vi "Mecanum Angular Drift Correction.vi"(1 "Reset":bool, 3 "Gyro":dbl, 6 "Joystick Rotation":dbl) -> (0 "Mecanum Rotation":dbl)   [LabVIEW 2014]
uses:
  <vilib>/addons/control/pid/pid.llb/PID (DBL).vi
  <vilib>/addons/control/pid/NI_PID_pid.lvlib
panel:
  in  "PID gains":T1={"proportional gain (Kc)"=1.0, "integral time (Ti, min)"=0.01, "derivative time (Td, min)"=0.0} {"derivative time (Td, min)" format="%.3f"; "integral time (Ti, min)" format="%.3f"; "proportional gain (Kc)" format="%.3f"}
  in  "Target Gyro Value":dbl
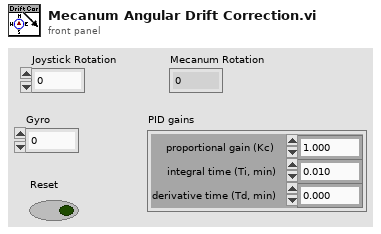
[diagram p1: front panel]
types:
  T1 = cluster{"proportional gain (Kc)":dbl, "integral time (Ti, min)":dbl, "derivative time (Td, min)":dbl}
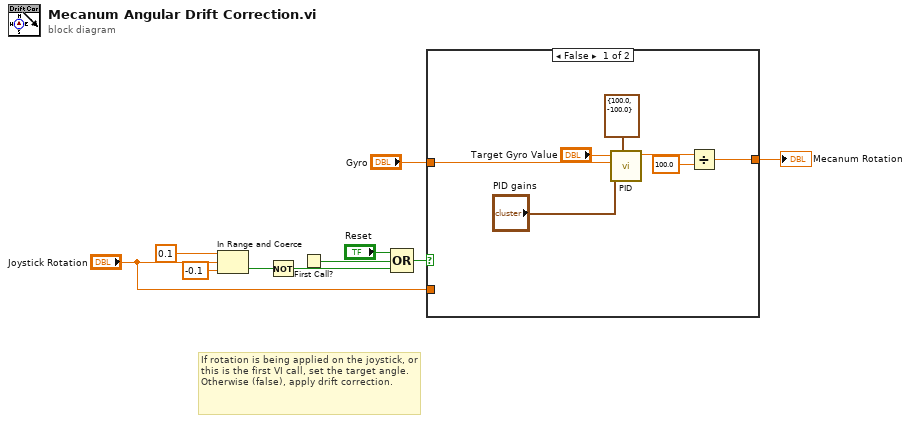
[diagram p0: block diagram]
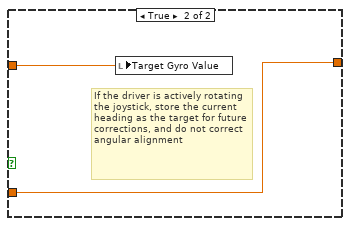
[diagram p2: hidden frame]
diagram:
  # "If rotation is being applied on the joystick, or this is the first VI call, set the target angle. Otherwise (false), apply drift correction."
  n1 = In Range and Coerce(upper limit=0.1 ("lower limit"), x="Joystick Rotation", lower limit=-0.1 ("upper limit")) -> (In Range?=w7:bool)  [unwired: 1 out]
  n2 = Not(x=w7) -> (.not. x?=w1:bool)
  n3 = First Call?() -> (First Call?: T/F=w2:bool)
  n4 = Compound Arithmetic op=OR("Reset", w2, w1) -> (w4:bool)
  n5 = case shown="False" w4 {
    tunnel: "Joystick Rotation" -> [_ w18]
    tunnel: "Gyro" -> [w17 w19]
    tunnel: [w12 w18] -> w5
    frame False {
      n6 = call-poly <vilib>:"PID.vi"("output range"=cluster{"output high":dbl, "output low":dbl} {"output high"=100.0, "output low"=-100.0}, "PID gains"="PID gains", "process variable"=w17, "setpoint"="Target Gyro Value") -> ("output"=w14:dbl)  [unwired: 6 in, 1 out]
      n7 = Divide(x=w14, y=100.0) -> (x/y=w12:dbl)
    }
    frame True {
      # "If the driver is actively rotating the joystick, store the current heading as the target for future corrections, and do not correct angular alignment"
      n8 = local write "Target Gyro Value"(w19) -> ()
    }
  }
  "Mecanum Rotation" <- w5
